vi "Read Barcodes (ARGB).vi"(7 "Options (Default)":refnum<class "ZXing.lvclass">, 8 "error in (no error)":errorcluster, 11 "ARGB Image in":T7) -> (0 "error out":errorcluster, 2 "Barcodes":T1[](array[typedef]) {"Error Type" items=["None", "Format", "Checksum", "Unsupported"]}, 3 "ARGB Image":T7)   [LabVIEW 2020, in "feature_detection.lvlib" / "ZXing.lvclass"]
doc: "Use the ZXing Barcode Reader to Detect Compatible Items in an Image."
uses:
  ZXing.lvclass
  image/ARGB Image.ctl
  Barcode.ctl
  Format.ctl
  Content Type.ctl
  common/Quad Corners.ctl
  common/Image Point (Float).ctl
  Error Type.ctl
  ZXing.lvclass/ZXing.ctl
  a90e4b0e-e65a-4d68-81f3-9c053758d966.vi
  <vilib>/Utility/error.llb/Error Cluster From Error Code.vi
  common/common.lvlib
  image/image.lvlib
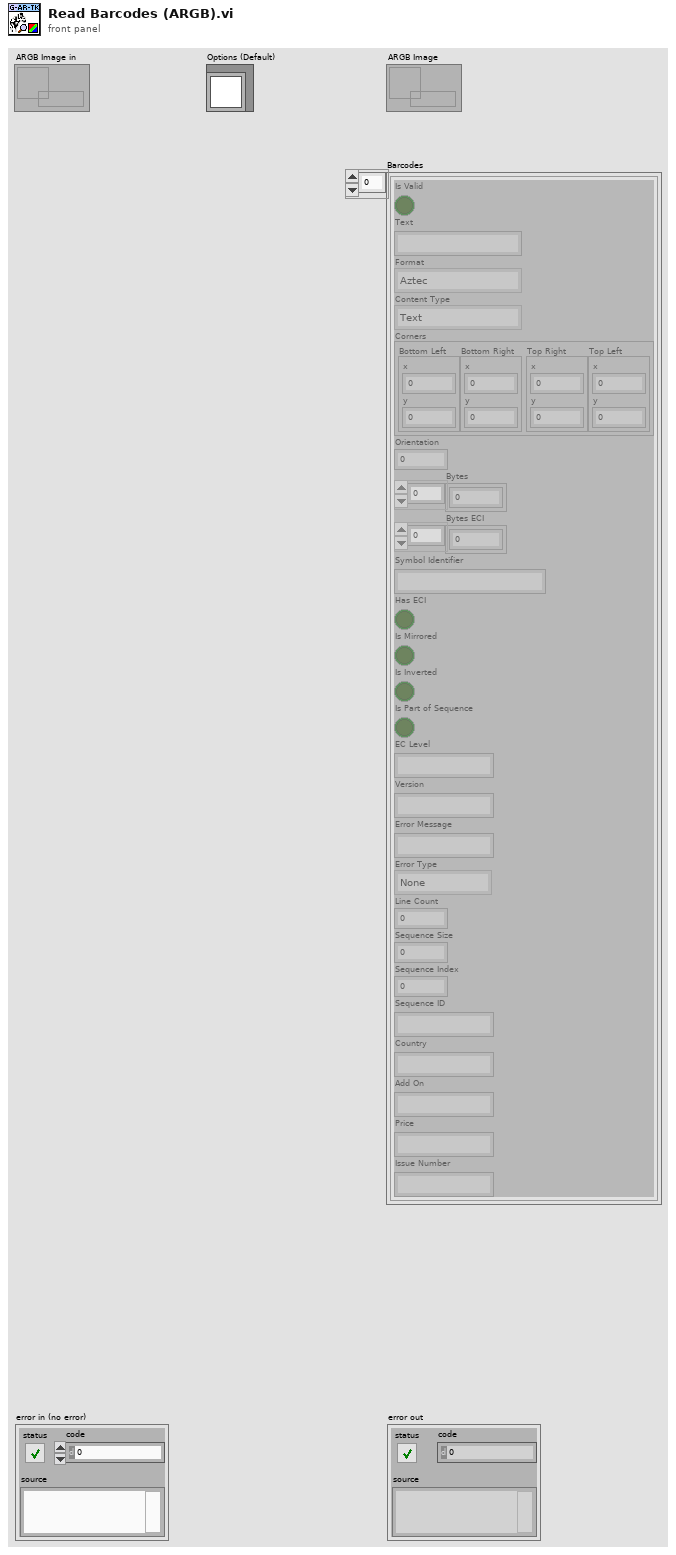
[diagram p1: front panel]
types:
  T1 = typedef "feature_detection.lvlib/ZXing.lvclass/Barcode.ctl" = cluster{"Is Valid":bool, "Text":string, "Format":T2, "Content Type":T3, "Corners":T4, "Orientation":i32, "Bytes":u8[], "Bytes ECI":u8[], "Symbol Identifier":string, "Has ECI":bool, "Is Mirrored":bool, "Is Inverted":bool, "Is Part of Sequence":bool, "EC Level":string, "Version":string, "Error Message":string, "Error Type":T6, "Line Count":i32, "Sequence Size":i32, "Sequence Index":i32, "Sequence ID":string, "Country":string, "Add On":string, "Price":string, "Issue Number":string}
  T2 = typedef "feature_detection.lvlib/ZXing.lvclass/Format.ctl" = enum8{"Aztec", "Codabar", "Code 39", "Code 93", "Code 128", "Data Bar", "Data Bar Expanded", "Data Matrix", "EAN 8", "EAN 13", "ITF", "Maxi Code", "PDF417", "QR Code", "UPCA", "UPCE", "Micro QR Code", "RM QR Code", "DX Film Edge", "Data Bar Limited"}
  T3 = typedef "feature_detection.lvlib/ZXing.lvclass/Content Type.ctl" = enum8{"Text", "Binary", "Mixed", "GS1", "ISO15434", "UnknownECI"}
  T4 = typedef "common.lvlib/Quad Corners.ctl" = cluster{"Bottom Left":T5, "Bottom Right":T5, "Top Right":T5, "Top Left":T5}
  T5 = typedef "common.lvlib/Image Point (Float).ctl" = cluster{"x":dbl, "y":dbl}
  T6 = typedef "feature_detection.lvlib/ZXing.lvclass/Error Type.ctl" = u8
  T7 = typedef "image.lvlib/ARGB Image.ctl" = refnum<data-value>
  T8 = typedef "feature_detection.lvlib/ZXing.lvclass/Options-Data.ctl" = cluster{"Try Harder":bool, "Try Rotate":bool, "Try Invert":bool, "Try Downscale":bool, "Is Pure":bool, "Try Code 39 Extended Mode":bool, "Return Errors":bool, "Downscale Factor":u8, "Min Line Count":u8, "Max Number of Symbols":u8, "Binarizer":T9, "EAN Add-On Symbol":T10, "Text Mode":T11, "Character Set":T12, "Downscale Threshold":u16, "Formats":T2[], "non_default_bit_flags":u16}
  T9 = typedef "feature_detection.lvlib/ZXing.lvclass/Binarizer.ctl" = enum8{"Local Average", "Global Histogram", "Fixed Threshold", "Bool Cast"}
  T10 = typedef "feature_detection.lvlib/ZXing.lvclass/EAN Add-On Symbol.ctl" = enum8{"Ignore", "Read", "Require"}
  T11 = typedef "feature_detection.lvlib/ZXing.lvclass/Text Mode.ctl" = enum8{"Plain", "ECI", "HRI", "Hex", "Escaped"}
  T12 = typedef "feature_detection.lvlib/ZXing.lvclass/Character Set.ctl" = enum8{"ASCII", "ISO8859_1", "ISO8859_2", "ISO8859_3", "ISO8859_4", "ISO8859_5", "ISO8859_6", "ISO8859_7", "ISO8859_8", "ISO8859_9", "ISO8859_10", "ISO8859_11", "ISO8859_13", "ISO8859_14", "ISO8859_15", "ISO8859_16", "Cp437", "Cp1250", "Cp1251", "Cp1252", "Cp1256", "Shift_JIS", "Big5", "GB2312", "GB18030", "EUC_JP", "EUC_KR", "UTF16BE", "UTF8", "UTF16LE", "UTF32BE", "UTF32LE", "BINARY"}
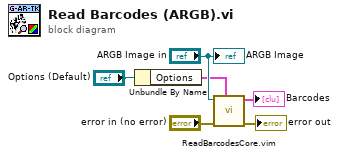
[diagram p0: block diagram]
diagram:
  n1 = Unbundle By Name("Options (Default)") -> ("Options"=w2:T8)
  n2 = call "ReadBarcodesCore.vim"("ZXing  in"=w2, "error in (no error)"="error in (no error)", "Greyscale Image in"="ARGB Image in") -> ("error out"=→"error out":errorcluster, "Barcodes"=→"Barcodes":T1[])  [unwired: 7 in]
  "ARGB Image" <- "ARGB Image in"
